vi "WPI_JoystickRefNum Registry Get.vi"(8 "error in (no error)":errorcluster, 10 "refnum name":string="My Joystick RefNum") -> (0 "error out":errorcluster, 3 "JoystickDevRef":T1={"Device"=enum."USB 1"})   [LabVIEW 2017]
doc: "Gets the reference you specify. You first must set the reference with the RefNum Registry Set VI."
uses:
  <vilib>/Rock Robotics/WPI/Joystick/WPI_JoystickDevRef.ctl
  <vilib>/Rock Robotics/WPI/Joystick/WPI_JoystickDeviceEnum.ctl
  <vilib>/Rock Robotics/WPI/Utilities/Refnum Registry Operation.ctl
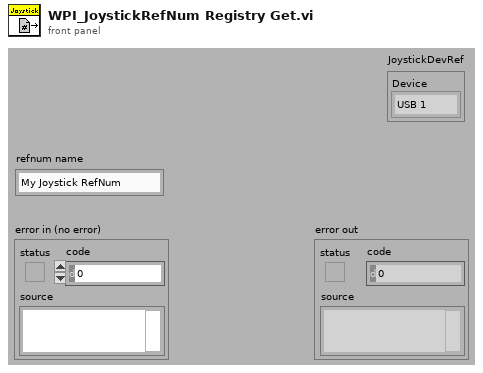
[diagram p1: front panel]
types:
  T1 = typedef "WPI_JoystickDevRef.ctl" = cluster{"Device":T2}
  T2 = typedef "WPI_JoystickDeviceEnum.ctl" = enum16{"USB 0", "USB 1", "USB 2", "USB 3", "USB 4", "USB 5"}
  T3 = typedef "Refnum Registry Operation.ctl" = enum16{"set", "get", "delete", "get all names", "read name"}
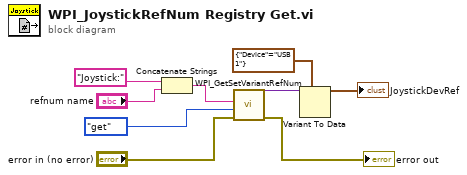
[diagram p0: block diagram]
diagram:
  n1 = Concatenate Strings("Joystick:", "refnum name") -> (w1:string)
  n2 = call <vilib>:"WPI_GetSetVariantRefNum.vi"("error in (no error)"="error in (no error)", "Operation"=Refnum_Registry_Operation."get" ("menu"), "refnum name"=w1) -> ("error out"=→"error out":errorcluster, "DevRef"=w6:variant)  [unwired: 6 in, 1 out]
  n3 = Variant To Data(type=T1 {"Device"=enum."USB 1"} ("JoystickDevRef"), Variant=w6) -> (data=→"JoystickDevRef":T1)  [unwired: 1 in, 1 out]
